vi "Set Angle.vi"(5 "Fine Tunning":dbl, 7 "Fine Tune?":bool, 9 "AIDeviceRef":T1, 10 "Angle":dbl) -> (0 "Current Angle(above Horizon)":dbl, 1 "Angle SET":bool, 2 "Angle Motor":dbl)   [LabVIEW 2011]
uses:
  <vilib>/Rock Robotics/WPI/AnalogChannel/WPI_AnalogChannelDevRef.ctl
  <vilib>/Rock Robotics/SystemInterfaces/Typedef/FPGA_TypedefAnalogModule.ctl
  <vilib>/Rock Robotics/SystemInterfaces/AI/FPGA_AIChannel.ctl
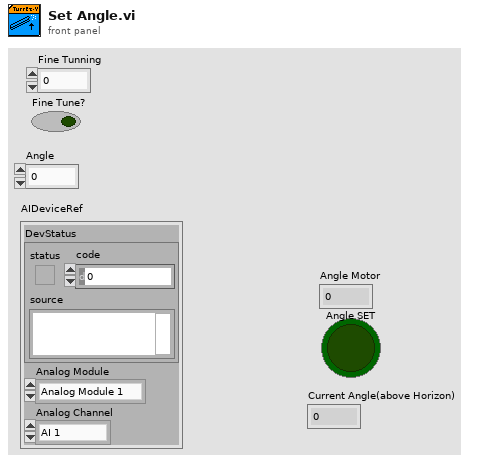
[diagram p1: front panel]
types:
  T1 = typedef "WPI_AnalogChannelDevRef.ctl" = cluster{"DevStatus":errorcluster, "Analog Module":T2, "Analog Channel":T3}
  T2 = typedef "FPGA_TypedefAnalogModule.ctl" = enum16{"Analog Module 1", "Analog Module 2"}
  T3 = typedef "FPGA_AIChannel.ctl" = enum8{"AI 1", "AI 2", "AI 3", "AI 4", "AI 5", "AI 6", "AI 7", "AI 8", "Invalid"}
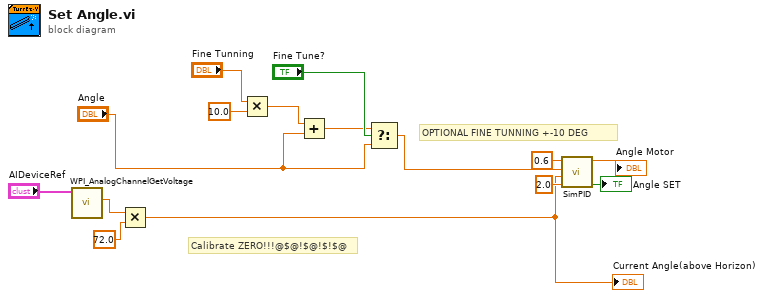
[diagram p0: block diagram]
diagram:
  # "OPTIONAL FINE TUNNING +-10 DEG"
  # "Calibrate ZERO!!!@$@!$@!$!$@"
  n1 = call <vilib>:"WPI_AnalogChannelGetVoltage.vi"("AIDeviceRef"="AIDeviceRef") -> ("Voltage"=w14:dbl)  [unwired: 8 in, 2 out]
  n2 = Multiply(x=w14, y=72.0 ("Voltage")) -> (x*y=w1:dbl)
  "Current Angle(above Horizon)" <- w1
  n3 = Multiply(x="Fine Tunning", y=10.0) -> (x*y=w8:dbl)
  n4 = Add(x=w8, y="Angle") -> (x+y=w10:dbl)
  n5 = Select(t=w10, s="Fine Tune?", f="Angle") -> (s? t:f=w11:dbl)
  n6 = call "SimPID.vi"("Range"=2.0, "Position"=w1, "Set Point"=w11, "Gain"=0.6) -> ("On Target"=→"Angle SET":bool, "result"=→"Angle Motor":dbl)  [unwired: 5 in]
